vi "Read ADC.vi"(8 "error in (no error)":errorcluster, 10 "ADC canal":dbl, 11 "NXP in":refnum<class "NXP.lvclass">) -> (0 "error out":errorcluster, 3 "NXP out":refnum<class "NXP.lvclass">)   [LabVIEW 2020, in "NXP.lvclass"]
doc: "Método heredado del padre con un override"
uses:
  NXP.lvclass
  78867b58-af9b-4f47-9d7e-921659e7fb04.vi
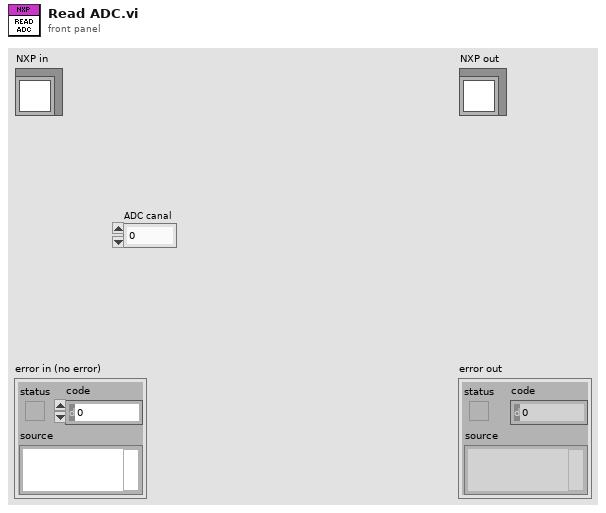
[diagram p1: front panel]
types:
  T1 = typedef "Serial device.lvclass/Brand combobox.ctl" = string
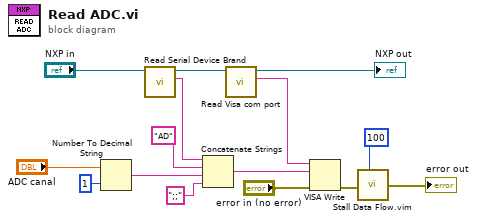
[diagram p0: block diagram]
diagram:
  n1 = Number To Decimal String(number="ADC canal", width (-)=i16 1) -> (decimal integer string=w9:string)
  n2 = call-dynamic "Read Serial Device Brand.vi"("Serial device in"="NXP in") -> ("Serial Device Brand"=w11:T1, "Serial device out"=w15:refnum<class "NXP.lvclass">)  [unwired: 8 in, 1 out]
  n3 = Concatenate Strings(w11, "AD" ("string"), w9, ";;" ("string")) -> (w6:string)
  n4 = call-dynamic "Read Visa com port.vi"("Serial device in"=w15) -> ("Visa com port"=w7:string, "Serial device out"=→"NXP out":refnum<class "NXP.lvclass">)  [unwired: 8 in, 1 out]
  n5 = VISA Write(VISA resource name=w7, write buffer=w6, error in (no error)="error in (no error)") -> (error out=w3:errorcluster)  [unwired: 2 out]
  n6 = call "Stall Data Flow.vim"("value in"=w3, "milliseconds to wait"=u32 100) -> ("value out"=→"error out":errorcluster)  [unwired: 1 out]
